vi "GapDetectionNew_nextFour_BM_markus_4_Ellipse.vi"(8 "Sigma in Prozent":dbl=3.0, 9 "Gap":dbl=85.0, 11 "Locations":dbl[](array[numeric])=[1075.5115609583977, 1096.8761989990003, 1148.4828033713086, 1170.9683288122183, 1215.5424277113636]) -> (1 "Wahrscheinlichkeit":dbl=9.225927080869098e-137, 2 "Gap":dbl=21.364638040602586, 3 "GapPresent":bool, 5 "t_1":dbl, 7 "t_2":dbl)   [LabVIEW 2014]
panel:
  in  "probaility higher than":dbl=0.9
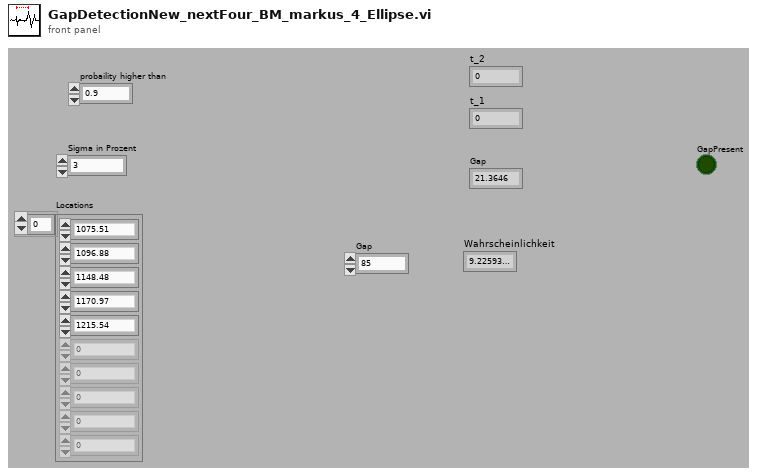
[diagram p1: front panel]
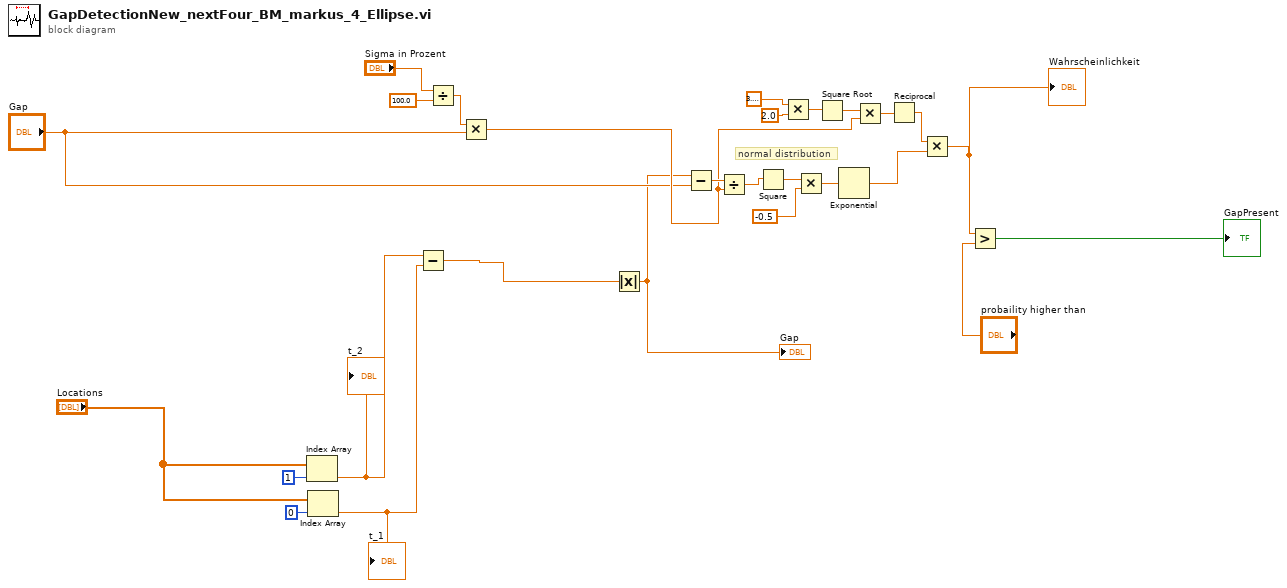
[diagram p0: block diagram]
diagram:
  # "normal distribution"
  n1 = Index Array(array="Locations", index=1) -> (element=w25:dbl)
  "t_2" <- w25
  n2 = Index Array(array="Locations", index=0) -> (element=w24:dbl)
  "t_1" <- w24
  n3 = Subtract(x=w25, y=w24) -> (x-y=w4:dbl)
  n4 = Divide(x="Sigma in Prozent", y=100.0) -> (x/y=w11:dbl)
  n5 = Multiply(x=w11, y="Gap") -> (x*y=w9:dbl)
  n6 = Absolute Value(x=w4) -> (abs(x)=w1:dbl)
  "Gap" <- w1
  n7 = Subtract(x=w1, y="Gap") -> (x-y=w18:dbl)
  n8 = Divide(x=w18, y=w9) -> (x/y=w17:dbl)
  n9 = Square(x=w17) -> (x^2=w16:dbl)
  n10 = Multiply(x=3.141592653589793, y=2.0) -> (x*y=w15:dbl)
  n11 = Multiply(x=w16, y=-0.5) -> (x*y=w22:dbl)
  n12 = Square Root(x=w15) -> (sqrt(x)=w14:dbl)
  n13 = Exponential(1:w22) -> (0:w5:dbl)
  n14 = Multiply(x=w14, y=w9) -> (x*y=w13:dbl)
  n15 = Reciprocal(x=w13) -> (1/x=w6:dbl)
  n16 = Multiply(x=w6, y=w5) -> (x*y=w3:dbl)
  "Wahrscheinlichkeit" <- w3
  n17 = Greater?(x=w3, y="probaility higher than") -> (0:→"GapPresent":bool)
